vi "Check and Get Sizes.vi"(8 "error in (no error)":errorcluster, 9 "test commands":string[](array[string]), 10 "variable name":string, 11 "GOLPI ref. in":T1={"pipe handle"={"lv_proc.dll file path"=path "", "process instance handle"=[]}, "fast read timeout [ms]"=500, "fast read settle time [ms]"=10, "fast read to multiple [ms]"=1, "max elements per input line"=100, "slow read timeout [ms]"=5000, "stdin double format specifier"="%_16e"}) -> (0 "error out":errorcluster, 1 "octave sizes":i32[](array[numeric]), 2 "all tests OK?":bool, 3 "GOLPI ref. out":T1={"pipe handle"={"lv_proc.dll file path"=path "", "process instance handle"=[]}, "fast read timeout [ms]"=500, "fast read settle time [ms]"=10, "fast read to multiple [ms]"=1, "max elements per input line"=100, "slow read timeout [ms]"=5000, "stdin double format specifier"="%_16e"})   [LabVIEW 2013, in "GOLPI library.lvlib"]
doc: "Checks GNU Octave variable and gets its size. 'variable name' is the name of the variable. 'test commands' is array of GNU Octave commands with boolean output applied to the variable. I.e. to read noncomplex double scalar variable 'x', following array should be supplied:\nisnumeric\nisscalar\n~isscomplex\nTests performed are:\nisnumeric(x)\nisscalar(x)\n~iscomplex(x)\nIf output of all tests is '1', output 'all tests OK?' is true.\nReturns size of variable in GNU Octave metric (i.e. no elements with zero indexes)"
uses:
  GOLPI library.lvlib
  Type Definitions/GOLPI reference Type Def.ctl
  LV Process.lvlibp/Pipe Handle.ctl
  Type Definitions/Custom Error Codes Enum Type Def.vi
  LV Process.lvlibp
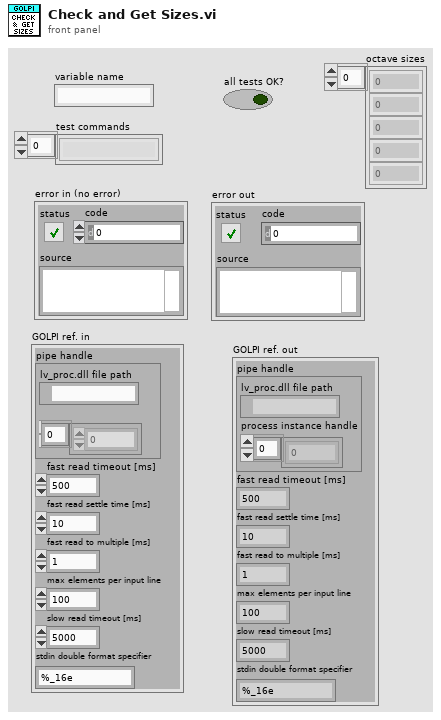
[diagram p1: front panel]
types:
  T1 = typedef "GOLPI library.lvlib/GOLPI reference Type Def.ctl" = cluster{"pipe handle":T2, "fast read timeout [ms]":u32, "fast read settle time [ms]":u32, "fast read to multiple [ms]":u32, "max elements per input line":u32, "slow read timeout [ms]":u32, "stdin double format specifier":string}
  T2 = typedef "LV Process.lvlibp/Pipe Handle.ctl" = cluster{"lv_proc.dll file path":path, "process instance handle":u32[]}
  T3 = typedef "GOLPI library.lvlib/Custom Error Codes Enum Type Def.vi" = enum16{"no error", "00 working directory PAR1 missing", "01 octave binary PAR1 missing", "02 octave report error PAR1", "03 empty output last cmd PAR1", "04 missing temporary file PAR1", "05 pwd PAR 1 not exist", "10 var PAR1 not string", "11 var PAR1 not num, scal, ~compl", "12 var PAR1 not num, scal, compl", "13 var PAR1 not num, vect, ~compl", "14 var PAR1 not num, vect, compl", "15 var PAR1 not num, mat, ~compl", "16 var PAR1 not num, mat, ~compl", "30 WARNING read timeout", "99 not finished"}
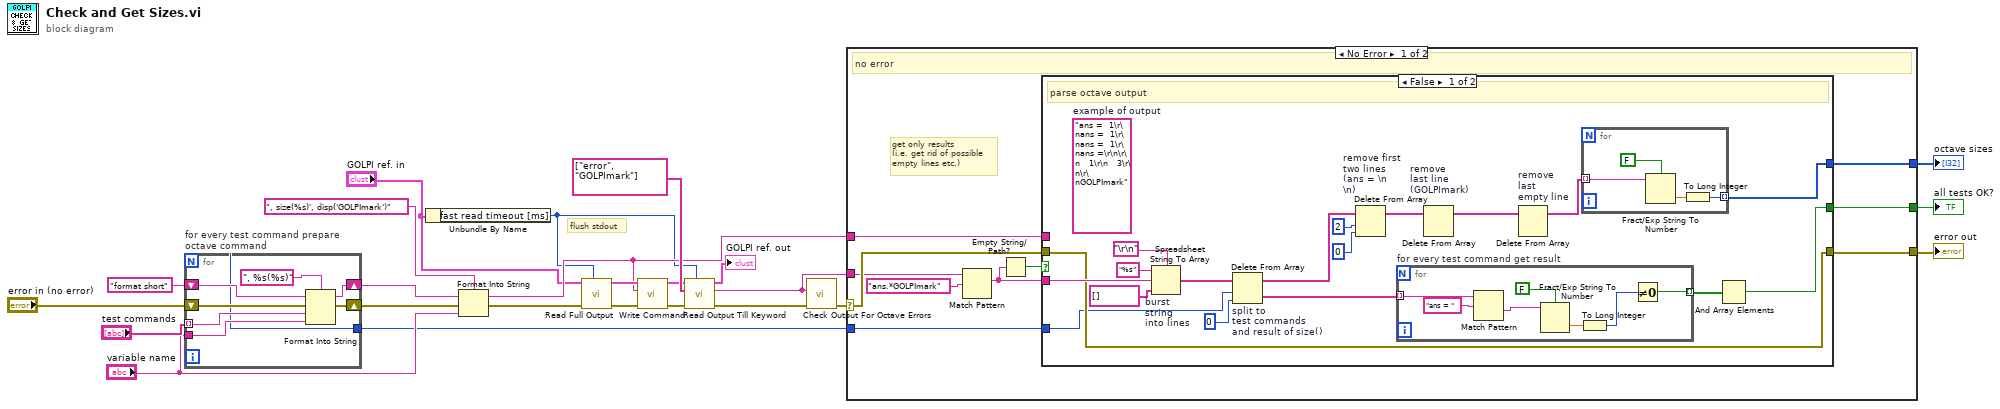
[diagram p0: block diagram]
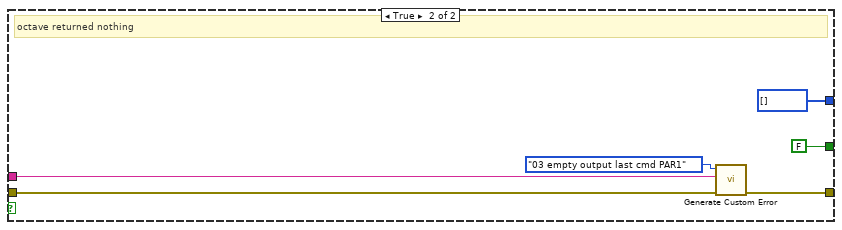
[diagram p2: hidden frame]
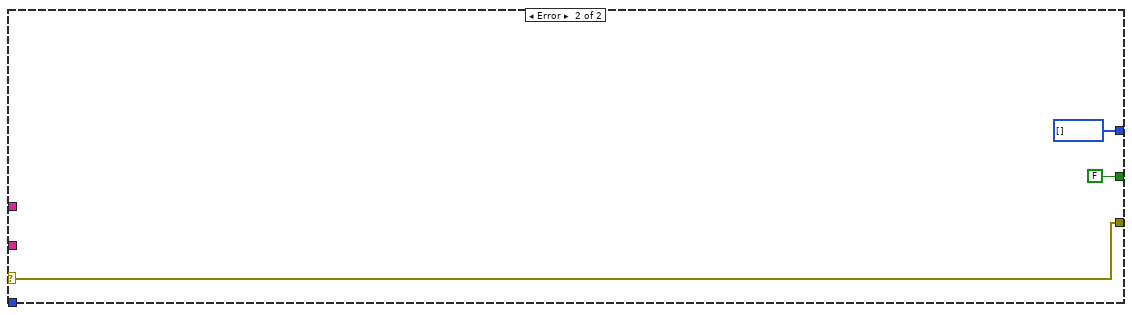
[diagram p3: hidden frame]
diagram:
  # "flush stdout"
  n1 = for "for every test command prepare\noctave command" {
    N -> [w25]
    tunnel: "test commands" -> [w30] mode=indexing
    tunnel: "variable name" -> [w29]
    shift-right: [w28] -> w18
    shift-left: "format short" -> [w31]
    shift-right: [w26] -> w19
    shift-left: "error in (no error)" -> [w27]
    tunnel: [w25] -> w4
    n2 = Format Into String(format string=", %s(%s)", initial string=w31, error in=w27, w30, w29) -> (resulting string=w28:string, error out=w26:errorcluster)
  }
  n3 = Unbundle By Name("GOLPI ref. in") -> ("fast read timeout [ms]"=w2:u32)
  n4 = Format Into String(format string=", size(%s)', disp('GOLPImark')", initial string=w18, error in=w19, "variable name") -> (resulting string=w5:string, error out=w15:errorcluster)
  n5 = call "Read Full Output.vi"("timeout [ms]"=w2, "error in"=w15, "GOLPI ref. in"="GOLPI ref. in") -> ("error out"=w14:errorcluster, "GOLPI ref. out"=w13:T1)  [unwired: 5 in, 2 out]
  n6 = call "Write Command.vi"("error in"=w14, "command"=w5, "GOLPI ref. in"=w13) -> ("error out"=w10:errorcluster, "GOLPI ref. out"=w11:T1)  [unwired: 7 in]
  n7 = call "Read Output Till Keyword.vi"("timeout [ms]"=w2, "error in"=w10, "keywords"=string[] ["error", "GOLPImark"], "GOLPI ref. in"=w11) -> ("error out"=w9:errorcluster, "read buffer"=w8:string, "GOLPI ref. out"=→"GOLPI ref. out":T1)  [unwired: 4 in, 1 out]
  n8 = call "Check Output For Octave Errors.vi"("error in"=w9, "read buffer"=w8) -> ("error out"=w7:errorcluster)  [unwired: 9 in]
  n9 = case shown="No Error" w7 {
    selector: w7 -> [w40 w78]
    tunnel: [w42 FALSE] -> w20
    tunnel: [w41 i32[] []] -> w16
    tunnel: w8 -> [w34 _]
    tunnel: [w38 w78] -> w6
    tunnel: w5 -> [w37 _]
    tunnel: w4 -> [w36 _]
    frame No Error {
      # "get only results\n(i.e. get rid of possible\nempty lines etc.)"
      # "no error"
      n10 = Match Pattern(string=w34, regular expression="ans.*GOLPImark") -> (match substring=w33:string)  [unwired: 1 in, 3 out]
      n11 = Empty String/Path?(string/path=w33) -> (empty?=w39:bool)
      n12 = case shown="False" w39 {
        tunnel: [w50 FALSE] -> w42
        tunnel: [w44 i32[] []] -> w41
        tunnel: w33 -> [w55 _]
        tunnel: w40 -> [w54 w74]
        tunnel: [w54 w73] -> w38
        tunnel: w37 -> [_ w72]
        tunnel: w36 -> [w53 _]
        frame False {
          (unwired) "ans =  1\r\nans =  1\r\nans =  1\r\nans =\r\n\r\n   1\r\n   3\r\n\r\nGOLPImark"  # example of output
          # "parse octave output"
          n13 = Spreadsheet String To Array "burst\nstring\ninto lines"(delimiter (Tab)="\r\n", format string="%s", spreadsheet string=w55, array type (2D Dbl)=string[] []) -> (array=w57:string[])
          n14 = Delete From Array "split to\ntest commands\nand result of size()"(array=w57, length=w53, index=0) -> (deleted portion=w52:string[], array with subset deleted=w49:string[])
          n15 = Delete From Array "remove first\ntwo lines\n(ans = \\n\n\\n)"(array=w49, length=2, index=0) -> (array with subset deleted=w46:string[])  [unwired: 1 out]
          n16 = for "for every test command get result" {
            tunnel: w52 -> [w71] mode=indexing
            tunnel: [w65] -> w51 mode=indexing
            n17 = Match Pattern(string=w71, regular expression="ans = ") -> (after substring=w67:string)  [unwired: 1 in, 3 out]
            n18 = Fract/Exp String To Number(use system decimal point (T)=FALSE, string=w67) -> (number=w68:dbl)  [unwired: 2 in, 1 out]
            n19 = To Long Integer(number=w68) -> (32bit integer=w69:i32)
            n20 = Not Equal To 0?(x=w69) -> (x != 0?=w65:bool)
          }
          n21 = Delete From Array "remove\nlast line\n(GOLPImark)"(array=w46) -> (array with subset deleted=w43:string[])  [unwired: 2 in, 1 out]
          n22 = Delete From Array "remove\nlast\nempty line"(array=w43) -> (array with subset deleted=w45:string[])  [unwired: 2 in, 1 out]
          n23 = for {
            tunnel: w45 -> [w62] mode=indexing
            tunnel: [w61] -> w44 mode=indexing
            n24 = Fract/Exp String To Number(use system decimal point (T)=FALSE, string=w62) -> (number=w64:dbl)  [unwired: 2 in, 1 out]
            n25 = To Long Integer(number=w64) -> (32bit integer=w61:i32)
          }
          n26 = And Array Elements(Boolean array=w51) -> (logical AND=w50:bool)
        }
        frame True {
          # "octave returned nothing"
          n27 = call "Generate Custom Error.vi"("error in"=w74, "PAR1"=w72, "GOLPI error"=Custom_Error_Codes_Enum_Type_Def.vi."03 empty output last cmd PAR1" ("Enum")) -> ("error out"=w73:errorcluster)  [unwired: 8 in]
        }
      }
    }
    frame Error {
    }
  }
  "all tests OK?" <- w20
  "octave sizes" <- w16
  "error out" <- w6
